vi "Untitled 1.vi"() -> ()   [LabVIEW 2017, in "labview-standard-library.lvlib"]
uses:
  <vilib>/vision/Image Controls.llb/IMAQ Image.ctl
  labview-standard-library.lvlib
panel:
  out "Image":T1(plugin-control)
  out "time between":dbl
  in  "Stop":bool
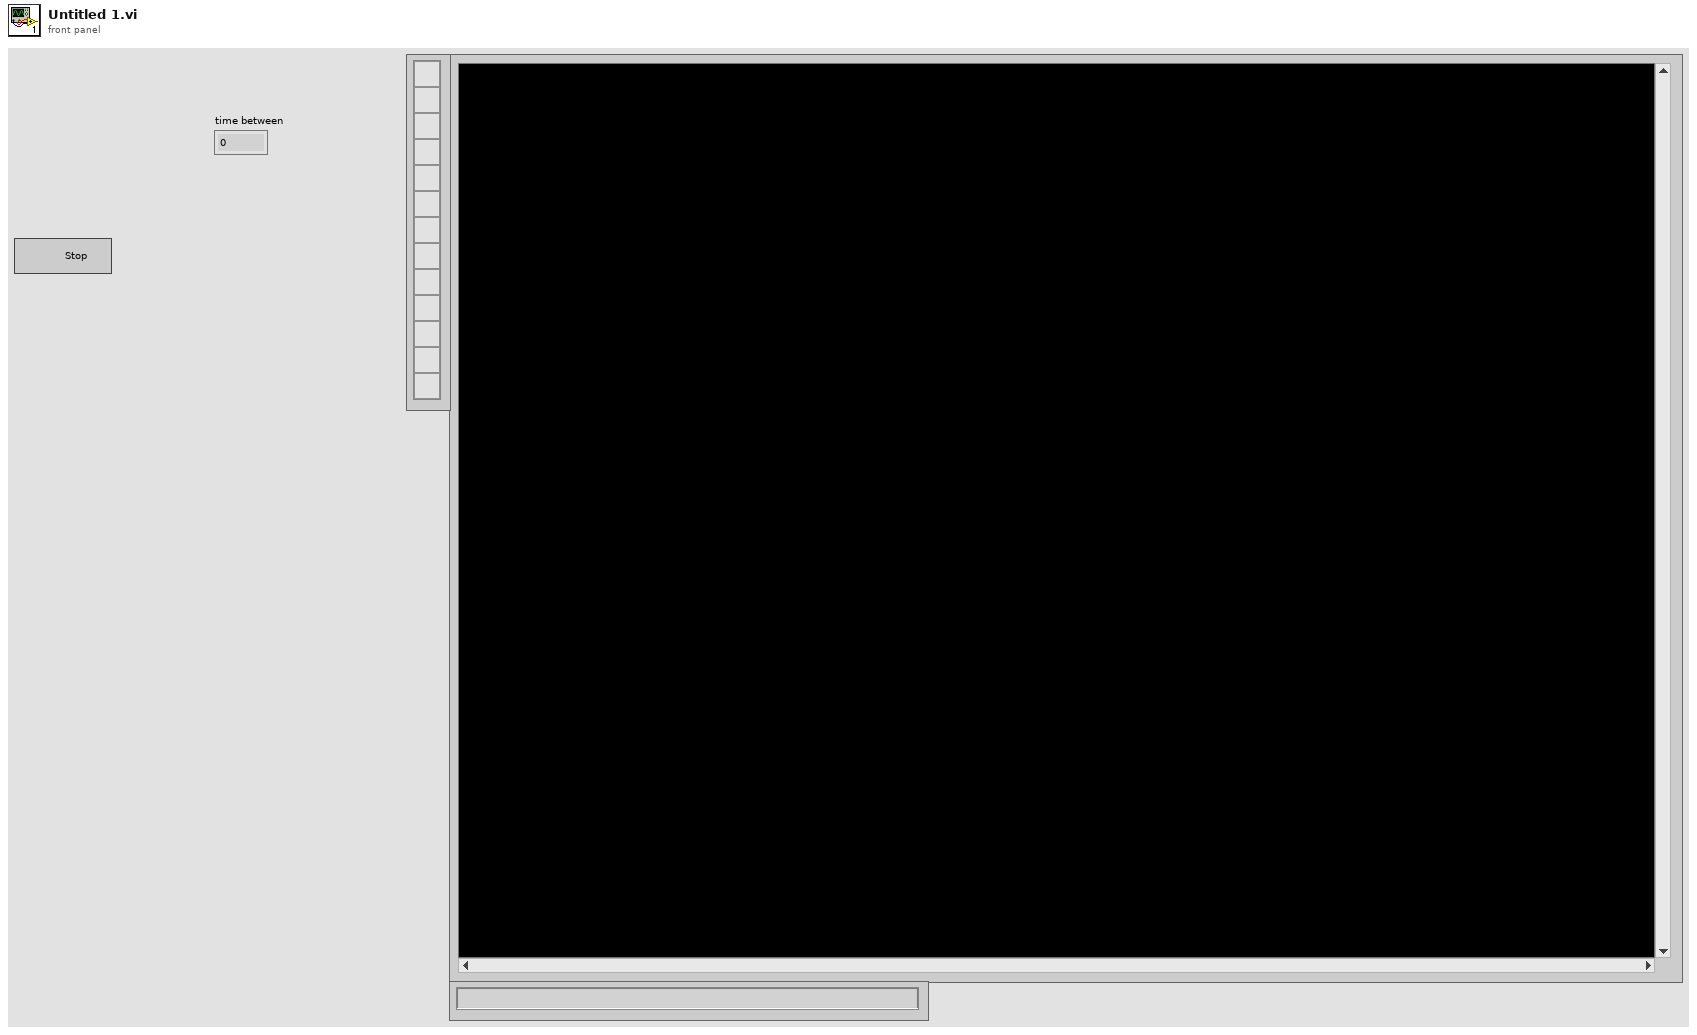
[diagram p1: front panel]
types:
  T1 = typedef "IMAQ Image.ctl" = refnum<image>
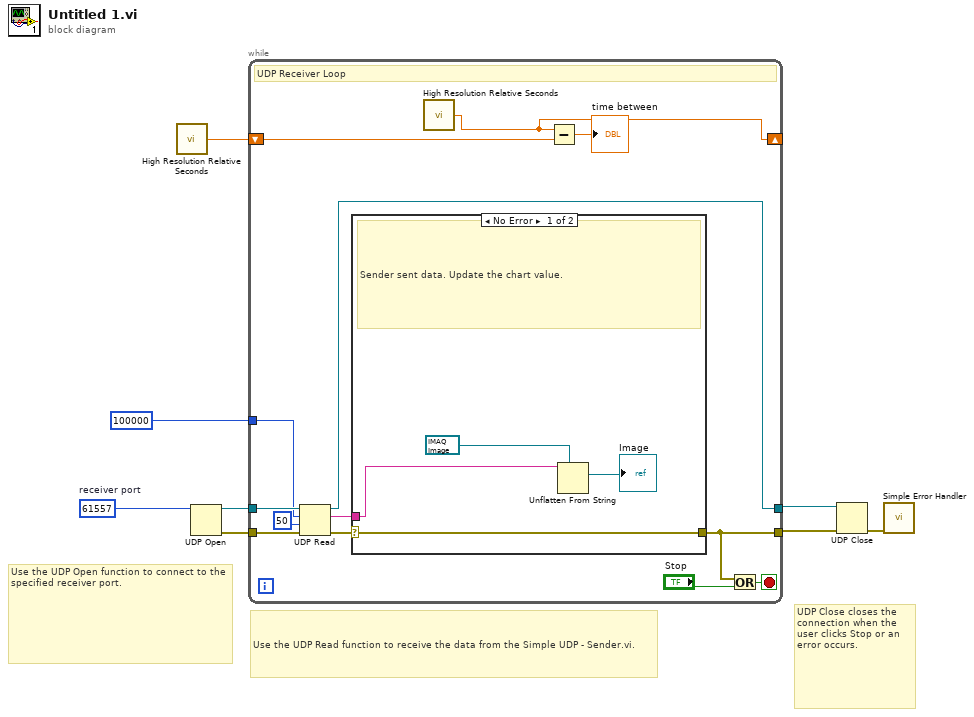
[diagram p0: block diagram]
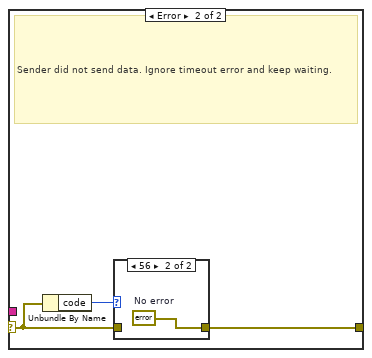
[diagram p2: hidden frame]
diagram:
  w3 = u16 61557  # receiver port
  # "UDP Close closes the connection when the user clicks Stop or an error occurs."
  # "Use the UDP Open function to connect to the specified receiver port."
  # "Use the UDP Read function to receive the data from the Simple UDP - Sender.vi."
  n1 = call <vilib>:"High Resolution Relative Seconds.vi"() -> ("relative seconds"=w2:dbl)
  n2 = UDP Open(11:w3) -> (port=w4:refnum<k16>, 0:w5:errorcluster)  [unwired: 4 in, 1 out]
  n3 = while {
    tunnel: w4 -> [w21]
    tunnel: [w13] -> w8
    tunnel: w5 -> [w18]
    tunnel: [w14] -> w6
    shift-right: [w12] -> _
    shift-left: w2 -> [w11]
    tunnel: 100000 ("max size (548)") -> [w9]
    stop <- w19 stop-if-true
    # "UDP Receiver Loop"
    n4 = UDP Read(connection ID=w21, max size (548)=w9, timeout ms (25000)=50, 8:w18) -> (data out=w16:string, error out=w15:errorcluster, 3:w13:refnum<k16>)  [unwired: 2 out]
    n5 = case shown="No Error" w15 {
      selector: w15 -> [w25 w27]
      tunnel: w16 -> [w24 _]
      tunnel: [w25 w26] -> w14
      frame No Error {
        # "Sender sent data. Update the chart value."
        n6 = Unflatten From String(type=T1 refnum ("New Image"), binary string=w24) -> (value=→"Image":T1)  [unwired: 3 in, 2 out]
      }
      frame Error {
        # "Sender did not send data. Ignore timeout error and keep waiting."
        n7 = Unbundle By Name(w27) -> ("code"=w28:i32)
        n8 = case shown="56" w28 {
          tunnel: w27 -> [w29 _]
          tunnel: [w29 w30] -> w26
          frame Default {
          }
          frame 56 {
            w30 = errorcluster {"status"=FALSE, "code"=0, "source"=""}  # No error
          }
        }
      }
    }
    n9 = call <vilib>:"High Resolution Relative Seconds.vi"() -> ("relative seconds"=w12:dbl)
    n10 = Subtract(x=w12, y=w11) -> (x-y=→"time between":dbl)
    n11 = Or(x=w14, y="Stop") -> (x .or. y?=w19:bool)
  }
  n12 = UDP Close(connection ID=w8, 8:w6) -> (error out=w7:errorcluster)  [unwired: 1 out]
  n13 = call <vilib>:"Simple Error Handler.vi"("error in (no error)"=w7) -> ()  [unwired: 1 in, 8 out]
